vi "Core-Wait.vi"(8 "error in (no error)":errorcluster, 11 "Engine in":refnum<class "Engine.lvclass">) -> (0 "error out":errorcluster, 3 "Engine out":refnum<class "Engine.lvclass">)   [LabVIEW 2020, in "GLF.lvlib" / "Engine.lvclass"]
uses:
  Engine.lvclass
  Engine.lvclass/Engine.ctl
  <vilib>/Saukko/LV SDL3/Sources/SDL3/Timer/Timer.lvlib
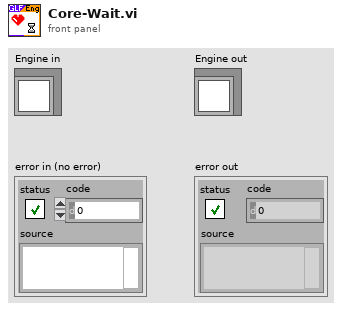
[diagram p1: front panel]
types:
  T1 = typedef "GLF.lvlib/Engine.lvclass/DVR--cluster.ctl" = cluster{"CMD Queue":T2, "Config":T3, "Ctxt":T5, "Metrics":T6, "Window Instances":map{T7, refnum<class "Window.lvclass">}, "Debug":T8}
  T2 = typedef "GLF.lvlib/Engine.lvclass/Command--queue.ctl" = refnum<queue>
  T3 = typedef "GLF.lvlib/Engine.lvclass/Config--cluster.ctl" = cluster{"Quit On Last Window Closed":bool, "VSync":T4, "FPS Target":dbl}
  T4 = typedef "GLF.lvlib/Engine.lvclass/VSync--enum.ctl" = enum16{"Disabled", "Enabled", "Adaptative"}
  T5 = typedef "GLF.lvlib/Engine.lvclass/Context--cluster.ctl" = cluster{"Ticks Begin":u64, "VSync Enabled":bool}
  T6 = typedef "GLF.lvlib/Engine.lvclass/Metrics--cluster.ctl" = cluster{"Uptime [ms]":u64, "Loop Time [ms]":u64, "Poll Events [ns]":u64, "Dequeue CMD [ns]":u64, "Update Layout [ns]":u64, "Render [ns]":u64}
  T7 = typedef "SDL3.lvlib/Video.lvlib/WindowID--integer.ctl" = u32
  T8 = typedef "GLF.lvlib/Engine.lvclass/Debug--cluster.ctl" = cluster{"Unhandled Events":map{T9, u64}}
  T9 = typedef "SDL3.lvlib/Events.lvlib/EventType--enum.ctl" = enum16{"LV_NONE", "LV_UNSUPPORTED", "SDL_EVENT_QUIT", "SDL_EVENT_LOCALE_CHANGED", "SDL_EVENT_SYSTEM_THEME_CHANGED", "SDL_EVENT_DISPLAY_ORIENTATION", "SDL_EVENT_DISPLAY_ADDED", "SDL_EVENT_DISPLAY_REMOVED", "SDL_EVENT_DISPLAY_MOVED", "SDL_EVENT_DISPLAY_DESKTOP_MODE_CHANGED", "SDL_EVENT_DISPLAY_CURRENT_MODE_CHANGED", "SDL_EVENT_DISPLAY_CONTENT_SCALE_CHANGED", "SDL_EVENT_WINDOW_SHOWN", "SDL_EVENT_WINDOW_HIDDEN", "SDL_EVENT_WINDOW_EXPOSED", "SDL_EVENT_WINDOW_MOVED", "SDL_EVENT_WINDOW_RESIZED", "SDL_EVENT_WINDOW_PIXEL_SIZE_CHANGED", "SDL_EVENT_WINDOW_METAL_VIEW_RESIZED", "SDL_EVENT_WINDOW_MINIMIZED", "SDL_EVENT_WINDOW_MAXIMIZED", "SDL_EVENT_WINDOW_RESTORED", "SDL_EVENT_WINDOW_MOUSE_ENTER", "SDL_EVENT_WINDOW_MOUSE_LEAVE", "SDL_EVENT_WINDOW_FOCUS_GAINED", "SDL_EVENT_WINDOW_FOCUS_LOST", "SDL_EVENT_WINDOW_CLOSE_REQUESTED", "SDL_EVENT_WINDOW_HIT_TEST", "SDL_EVENT_WINDOW_ICCPROF_CHANGED", "SDL_EVENT_WINDOW_DISPLAY_CHANGED", "SDL_EVENT_WINDOW_DISPLAY_SCALE_CHANGED", "SDL_EVENT_WINDOW_SAFE_AREA_CHANGED", "SDL_EVENT_WINDOW_OCCLUDED", "SDL_EVENT_WINDOW_ENTER_FULLSCREEN", "SDL_EVENT_WINDOW_LEAVE_FULLSCREEN", "SDL_EVENT_WINDOW_DESTROYED", "SDL_EVENT_WINDOW_HDR_STATE_CHANGED", "SDL_EVENT_KEY_DOWN", "SDL_EVENT_KEY_UP", "SDL_EVENT_TEXT_EDITING", "SDL_EVENT_TEXT_INPUT", "SDL_EVENT_KEYMAP_CHANGED", "SDL_EVENT_KEYBOARD_ADDED", "SDL_EVENT_KEYBOARD_REMOVED", "SDL_EVENT_TEXT_EDITING_CANDIDATES", "SDL_EVENT_MOUSE_MOTION", "SDL_EVENT_MOUSE_BUTTON_DOWN", "SDL_EVENT_MOUSE_BUTTON_UP", "SDL_EVENT_MOUSE_WHEEL", "SDL_EVENT_MOUSE_ADDED", "SDL_EVENT_MOUSE_REMOVED", "SDL_EVENT_JOYSTICK_AXIS_MOTION", "SDL_EVENT_JOYSTICK_BALL_MOTION", "SDL_EVENT_JOYSTICK_HAT_MOTION", "SDL_EVENT_JOYSTICK_BUTTON_DOWN", "SDL_EVENT_JOYSTICK_BUTTON_UP", "SDL_EVENT_JOYSTICK_ADDED", "SDL_EVENT_JOYSTICK_REMOVED", "SDL_EVENT_JOYSTICK_BATTERY_UPDATED", "SDL_EVENT_JOYSTICK_UPDATE_COMPLETE", "SDL_EVENT_GAMEPAD_AXIS_MOTION", "SDL_EVENT_GAMEPAD_BUTTON_DOWN", "SDL_EVENT_GAMEPAD_BUTTON_UP", "SDL_EVENT_GAMEPAD_ADDED", "SDL_EVENT_GAMEPAD_REMOVED", "SDL_EVENT_GAMEPAD_REMAPPED", "SDL_EVENT_GAMEPAD_TOUCHPAD_DOWN", "SDL_EVENT_GAMEPAD_TOUCHPAD_MOTION", "SDL_EVENT_GAMEPAD_TOUCHPAD_UP", "SDL_EVENT_GAMEPAD_SENSOR_UPDATE", "SDL_EVENT_GAMEPAD_UPDATE_COMPLETE", "SDL_EVENT_GAMEPAD_STEAM_HANDLE_UPDATED", "SDL_EVENT_FINGER_DOWN", "SDL_EVENT_FINGER_UP", "SDL_EVENT_FINGER_MOTION", "SDL_EVENT_CLIPBOARD_UPDATE", "SDL_EVENT_DROP_FILE", "SDL_EVENT_DROP_TEXT", "SDL_EVENT_DROP_BEGIN", "SDL_EVENT_DROP_COMPLETE", "SDL_EVENT_DROP_POSITION", "SDL_EVENT_AUDIO_DEVICE_ADDED", "SDL_EVENT_AUDIO_DEVICE_REMOVED", "SDL_EVENT_AUDIO_DEVICE_FORMAT_CHANGED", "SDL_EVENT_SENSOR_UPDATE", "SDL_EVENT_PEN_PROXIMITY_IN", "SDL_EVENT_PEN_PROXIMITY_OUT", "SDL_EVENT_PEN_DOWN", "SDL_EVENT_PEN_UP", "SDL_EVENT_PEN_BUTTON_DOWN", "SDL_EVENT_PEN_BUTTON_UP", "SDL_EVENT_PEN_MOTION", "SDL_EVENT_PEN_AXIS", "SDL_EVENT_CAMERA_DEVICE_ADDED", "SDL_EVENT_CAMERA_DEVICE_REMOVED", "SDL_EVENT_CAMERA_DEVICE_APPROVED", "SDL_EVENT_CAMERA_DEVICE_DENIED", "SDL_EVENT_RENDER_TARGETS_RESET", "SDL_EVENT_RENDER_DEVICE_RESET", "SDL_EVENT_POLL_SENTINEL", "SDL_EVENT_USER"}
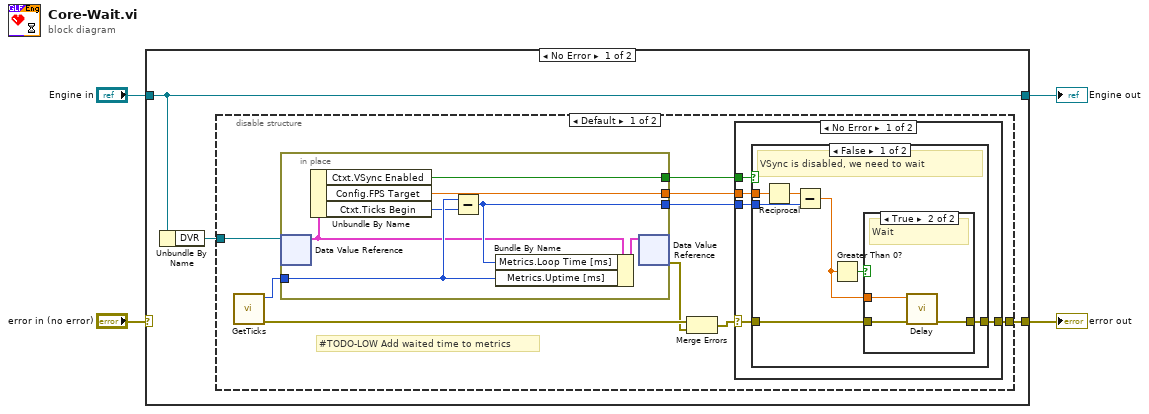
[diagram p0: block diagram]
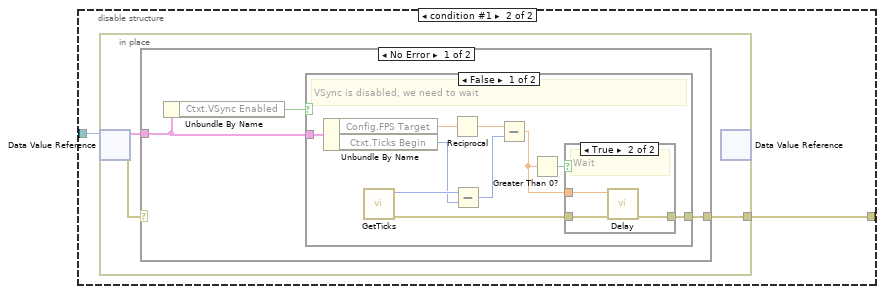
[diagram p5: hidden frame]
diagram:
  n1 = case shown="No Error" "error in (no error)" {
    selector: "error in (no error)" -> [_ w65]
    tunnel: [w6 w65] -> w4
    tunnel: "Engine in" -> [w7 w66]
    tunnel: [w7 w66] -> w1
    frame No Error {
      n2 = Unbundle By Name(w7) -> ("DVR"=w5:refnum<data-value>)
      n3 = disable-structure shown="Default" {
        disable-tunnel: [w16 w43] -> w6
        disable-tunnel: w5 -> [w15 w42]
        frame condition #0 (active) {
          # "#TODO-LOW Add waited time to metrics"
          n4 = call <vilib>:"GetTicks.vi"() -> ("error out"=w10:errorcluster, "Ticks [ms]"=w14:u64)  [unwired: 10 in]
          n5 = in-place {
            in-place-border: w14 -> [w22]
            in-place-border: [w21] -> w13
            in-place-border: [w19] -> w12
            in-place-border: [w18] -> w11
            n6 = in-place-dvr #1(w15) -> (w20:T1)  [unwired: 1 out]
            n7 = Unbundle By Name(w20) -> ("Ctxt.VSync Enabled"=w19:bool, "Config.FPS Target"=w18:dbl, "Ctxt.Ticks Begin"=w17:u64)
            n8 = Subtract(x=w22, y=w17) -> (x-y=w21:u64)
            n9 = Bundle By Name(cluster=w20, "Metrics.Loop Time [ms]"=w21, "Metrics.Uptime [ms]"=w22) -> (w23:T1)
            n10 = in-place-dvr #1(w23) -> (w8:errorcluster)  [unwired: 1 out]
          }
          n11 = Merge Errors(w10, w8) -> (w9:errorcluster)
          n12 = case shown="No Error" w9 {
            selector: w9 -> [w24 w41]
            tunnel: [w28 w41] -> w16
            tunnel: w13 -> [w27 _]
            tunnel: w12 -> [w26 _]
            tunnel: w11 -> [w25 _]
            frame No Error {
              n13 = case shown="False" w26 {
                tunnel: w24 -> [w31 w40]
                tunnel: [w34 w40] -> w28
                tunnel: w27 -> [w29 _]
                tunnel: w25 -> [w30 _]
                frame False {
                  # "VSync is disabled, we need to wait"
                  n14 = Reciprocal(x=w30) -> (1/x=w35:dbl)
                  n15 = Subtract(x=w35, y=w29) -> (x-y=w33:dbl)
                  n16 = Greater Than 0?(x=w33) -> (x > 0?=w32:bool)
                  n17 = case shown="True" w32 {
                    tunnel: w31 -> [w36 w39]
                    tunnel: [w36 w38] -> w34
                    tunnel: w33 -> [_ w37]
                    frame False {
                      # "Late"
                    }
                    frame True {
                      # "Wait"
                      n18 = call <vilib>:"Delay.vi"("No Error"=w39, "ms"=w37) -> ("error out"=w38:errorcluster)  [unwired: 9 in]
                    }
                  }
                }
                frame True {
                  # "No need to wait, this is done with the render present function"
                }
              }
            }
            frame Error {
            }
          }
        }
        frame condition #1 {
          n19 = in-place {
            in-place-border: [w46] -> w43
            n20 = in-place-dvr #2(w42) -> (w45:T1, w44:errorcluster)
            n21 = case shown="No Error" w44 {
              selector: w44 -> [_ w64]
              tunnel: [w48 w64] -> w46
              tunnel: w45 -> [w47 _]
              frame No Error {
                n22 = Unbundle By Name(w47) -> ("Ctxt.VSync Enabled"=w49:bool)
                n23 = case shown="False" w49 {
                  tunnel: [w57 _] -> w48
                  tunnel: w47 -> [w54 _]
                  frame False {
                    # "VSync is disabled, we need to wait"
                    n24 = Unbundle By Name(w54) -> ("Config.FPS Target"=w59:dbl, "Ctxt.Ticks Begin"=w51:u64)
                    n25 = call <vilib>:"GetTicks.vi"() -> ("error out"=w53:errorcluster, "Ticks [ms]"=w52:u64)  [unwired: 10 in]
                    n26 = Reciprocal(x=w59) -> (1/x=w58:dbl)
                    n27 = Subtract(x=w52, y=w51) -> (x-y=w50:u64)
                    n28 = Subtract(x=w58, y=w50) -> (x-y=w56:dbl)
                    n29 = Greater Than 0?(x=w56) -> (x > 0?=w55:bool)
                    n30 = case shown="True" w55 {
                      tunnel: w53 -> [w60 w63]
                      tunnel: [w60 w62] -> w57
                      tunnel: w56 -> [_ w61]
                      frame False {
                        # "Late"
                      }
                      frame True {
                        # "Wait"
                        n31 = call <vilib>:"Delay.vi"("No Error"=w63, "ms"=w61) -> ("error out"=w62:errorcluster)  [unwired: 9 in]
                      }
                    }
                  }
                  frame True {
                    # "No need to wait, this is done with the render present function"
                  }
                }
              }
              frame Error {
              }
            }
            n32 = in-place-dvr #2() -> ()  [unwired: 1 in, 2 out]
          }
        }
      }
    }
    frame Error {
    }
  }
  "error out" <- w4
  "Engine out" <- w1
